vi "TemperatureHumidityMonitor.vi"() -> ()   [LabVIEW 2013]
uses:
  InstrControl/ArduinoControl/ArduinoControl.lvclass
  InstrControl/InstrumentSetup.vi
  InstrControl/InstrControl.lvclass
panel:
  in  "VISA address":refnum<visa-resource-name>="COM24"
  in  "Duration":u32=43200 step=3600 format="%<%H:%M:%S>t"
  in  "Run":bool
  in  "quit":bool
  out "Run time":u32 format="%<%H:%M:%S>t"
  out "Humidity":dbl caption="Humidity [%]"
  out "Temp.":dbl caption="Temp. [°C]"
  in  "Interval [s]":u32=10
  out "Tgraph":cluster{u32[], dbl[]}[](graph)
  # "Temperature & Humidity Monitor"
  # "University of\nCambridge"
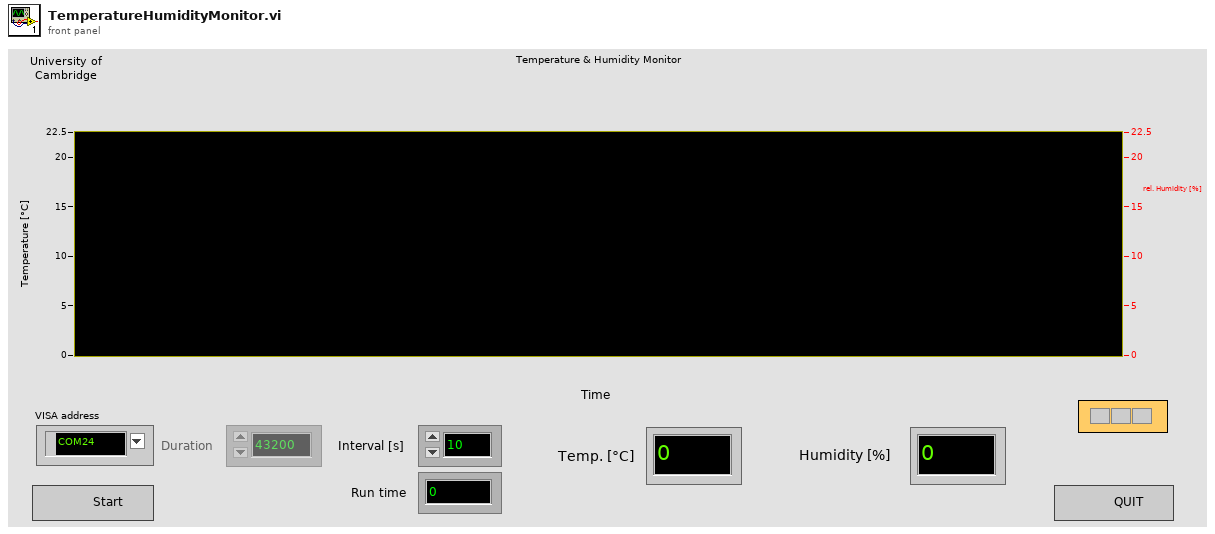
[diagram p1: front panel]
types:
  T1 = cluster{"VISA address":refnum<visa-resource-name>, "T sensor":enum16{"SHT", "DS"}, "Arduino":refnum<class "ArduinoControl.lvclass">}
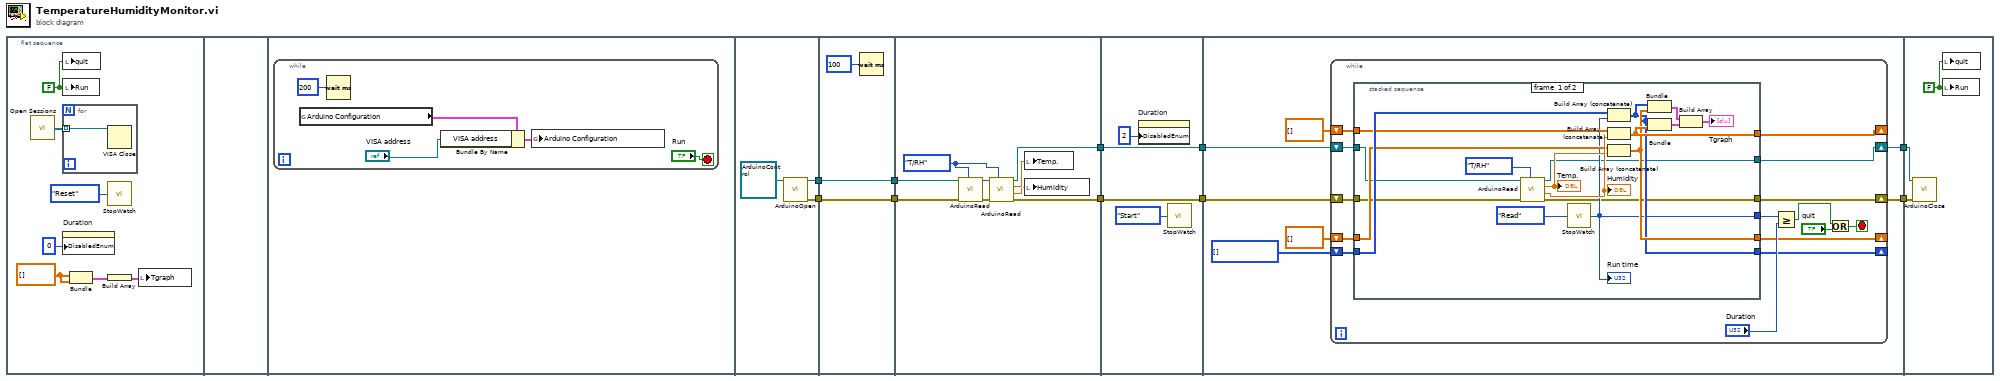
[diagram p0: block diagram]
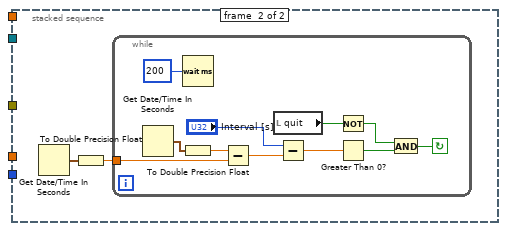
[diagram p2: hidden frame]
diagram:
  n1 = flat-sequence {
    tunnel: [w25] -> w4
    tunnel: [w24] -> w2
    tunnel: w4 -> [w29]
    tunnel: [w29] -> w3
    tunnel: w2 -> [w28]
    tunnel: [w28] -> w1
    tunnel: [w33] -> w6
    tunnel: [w32] -> w5
    tunnel: w3 -> [w31]
    tunnel: w1 -> [w30]
    tunnel: [w40] -> w10
    tunnel: [w39] -> w8
    tunnel: w6 -> [w39]
    tunnel: w5 -> [w40]
    tunnel: w10 -> [w46]
    tunnel: [w45] -> w9
    tunnel: w8 -> [w44]
    tunnel: [w43] -> w7
    tunnel: w9 -> [w97]
    tunnel: w7 -> [w96]
    frame #0 {
      w15 = dbl[] []
      w16 = FALSE
      n2 = call <vilib>:"Open Sessions.vi"() -> ("Array of Refnums"=w11:refnum<visa-resource-name>[])  [unwired: 2 in]
      n3 = local write "quit"(w16) -> ()
      n4 = local write "Run"(w16) -> ()
      n5 = for {
        tunnel: w11 -> [w18] mode=indexing
        n6 = VISA Close(VISA resource name=w18) -> ()  [unwired: 1 in, 1 out]
      }
      n7 = property on="Duration" class="DigNum (strict)"("DisabledEnum"=0) -> ()  [unwired: 2 in, 2 out]
      n8 = Bundle(w15, w15) -> (w13:cluster{dbl[], dbl[]})  [unwired: 1 in]
      n9 = call "StopWatch.vi"("Action"=enum16{"Start", "Stop", "Read", "Reset"}."Reset") -> ()  [unwired: 5 out]
      n10 = Build Array(w13) -> (w14:cluster{dbl[], dbl[]}[])
      n11 = local write "Tgraph"(w14) -> ()
    }
    frame #1 {
    }
    frame #2 {
      n12 = while {
        stop <- "Run" stop-if-true
        n13 = global read "InstrumentSetup.vi" "Arduino Configuration"() -> (w19:T1)
        n14 = Wait (ms)(milliseconds to wait=u32 200) -> ()  [unwired: 1 out]
        n15 = Bundle By Name(cluster=w19, "VISA address"="VISA address") -> (w21:T1)
        n16 = global write "InstrumentSetup.vi" "Arduino Configuration"(w21) -> ()
      }
    }
    frame #3 {
      n17 = call "ArduinoOpen.vi"("ArduinoControl in"=refnum<class "ArduinoControl.lvclass"> refnum) -> ("error out"=w24:errorcluster, "ArduinoControl out"=w25:refnum<class "ArduinoControl.lvclass">)  [unwired: 9 in]
    }
    frame #4 {
      n18 = Wait (ms)(milliseconds to wait=100) -> ()  [unwired: 1 out]
    }
    frame #5 {
      w38 = enum16{"T/RH", "Interlock", "Edgesense"}."T/RH" ("Arduino function")
      n19 = call "ArduinoRead.vi"("Arduino function"=w38, "error in (no error)"=w30, "ArduinoControl in"=w31) -> ("error out"=w37:errorcluster, "ArduinoControl out"=w36:refnum<class "ArduinoControl.lvclass">)  [unwired: 3 in, 4 out]
      n20 = call "ArduinoRead.vi"("Arduino function"=w38, "error in (no error)"=w37, "ArduinoControl in"=w36) -> ("error out"=w33:errorcluster, "rel. Humidity [%]"=w34:dbl, "Temperature [°C]"=w35:dbl, "ArduinoControl out"=w32:refnum<class "ArduinoControl.lvclass">)  [unwired: 3 in, 2 out]
      n21 = local write "Temp."(w35) -> ()
      n22 = local write "Humidity"(w34) -> ()
    }
    frame #6 {
      n23 = property on="Duration" class="DigNum (strict)"("DisabledEnum"=2) -> ()  [unwired: 2 in, 2 out]
      n24 = call "StopWatch.vi"("Action"=enum16{"Start", "Stop", "Read", "Reset"}."Start") -> ()  [unwired: 5 out]
    }
    frame #7 {
      n25 = while {
        shift-right: [w59] -> _
        shift-left: u32[] [] -> [w60]
        shift-right: [w55] -> _
        shift-left: dbl[] [] -> [w58]
        shift-right: [w56] -> _
        shift-left: dbl[] [] -> [w57]
        shift-right: [w52] -> w45
        shift-left: w46 -> [w53]
        shift-right: [w50] -> w43
        shift-left: w44 -> [w51]
        stop <- w61 stop-if-true
        n26 = stacked-sequence {
          tunnel: w60 -> [w81 _]
          tunnel: [w74 _] -> w59
          tunnel: w58 -> [w78 _]
          tunnel: w57 -> [w77 _]
          tunnel: [w76 _] -> w56
          tunnel: [w75 _] -> w55
          tunnel: [w70 _] -> w54
          tunnel: w53 -> [w69 _]
          tunnel: [w68 _] -> w52
          tunnel: w51 -> [w67 _]
          tunnel: [w66 _] -> w50
          frame #0 {
            n27 = call "ArduinoRead.vi"("Arduino function"=enum16{"T/RH", "Interlock", "Edgesense"}."T/RH", "error in (no error)"=w67, "ArduinoControl in"=w69) -> ("error out"=w66:errorcluster, "rel. Humidity [%]"=w80:dbl, "Temperature [°C]"=w79:dbl, "ArduinoControl out"=w68:refnum<class "ArduinoControl.lvclass">)  [unwired: 3 in, 2 out]
            "Humidity" <- w80
            "Temp." <- w79
            n28 = call "StopWatch.vi"("Action"=enum16{"Start", "Stop", "Read", "Reset"}."Read") -> ("Time elapsed"=w70:u32)  [unwired: 4 out]
            "Run time" <- w70
            n29 = Build Array (concatenate)(w81, w70) -> (w74:u32[])
            n30 = Build Array (concatenate)(w77, w80) -> (w76:dbl[])
            n31 = Build Array (concatenate)(w78, w79) -> (w75:dbl[])
            n32 = Bundle(w74, w75) -> (w73:cluster{u32[], dbl[]})  [unwired: 1 in]
            n33 = Bundle(w74, w76) -> (w72:cluster{u32[], dbl[]})  [unwired: 1 in]
            n34 = Build Array(w73, w72) -> (→"Tgraph":cluster{u32[], dbl[]}[])
          }
          frame #1 {
            n35 = Get Date/Time In Seconds() -> (seconds since 1Jan1904=w84:timestamp)
            n36 = To Double Precision Float(number=w84) -> (double precision float=w83:dbl)
            n37 = while {
              tunnel: w83 -> [w92]
              stop <- w85 continue-if-true
              n38 = Get Date/Time In Seconds() -> (seconds since 1Jan1904=w94:timestamp)
              n39 = Wait (ms)(milliseconds to wait=u32 200) -> ()  [unwired: 1 out]
              n40 = To Double Precision Float(number=w94) -> (double precision float=w93:dbl)
              n41 = Subtract(x=w93, y=w92) -> (x-y=w91:dbl)
              n42 = local read "quit"() -> (w88:bool)
              n43 = Subtract(x="Interval [s]", y=w91) -> (x-y=w89:dbl)
              n44 = Not(x=w88) -> (.not. x?=w87:bool)
              n45 = Greater Than 0?(x=w89) -> (x > 0?=w86:bool)
              n46 = And(x=w87, y=w86) -> (x .and. y?=w85:bool)
            }
          }
        }
        n47 = Greater Or Equal?(x=w54, y="Duration") -> (x >= y?=w62:bool)
        n48 = Or(x=w62, y="quit") -> (x .or. y?=w61:bool)
      }
    }
    frame #8 {
      w98 = FALSE
      n49 = call "ArduinoClose.vi"("error in (no error)"=w96, "ArduinoControl in"=w97) -> ()  [unwired: 8 in, 2 out]
      n50 = local write "quit"(w98) -> ()
      n51 = local write "Run"(w98) -> ()
    }
  }
